vi "GEA2 Script_Parse ERD Read.vi"(0 "Data":string, 11 "Error In":errorcluster) -> (2 "Expected Responses":string[](array[string]), 4 "GEA Inputs":T1 {"Destination" format="%.0x"; "Source" format="%.0x"}, 8 "Read ERD List":T2(array[cluster]) {"ERD Number" format="%.0x"}, 15 "Error Out":errorcluster)   [LabVIEW 2023]
uses:
  LabVIEW GEA2 Toolkit/GEA3/type defs/Source_Destination.ctl
  LabVIEW GEA2 Toolkit/GEA3/type defs/ERD Read Data In.ctl
  <vilib>/regexp/Match Regular Expression.xnode
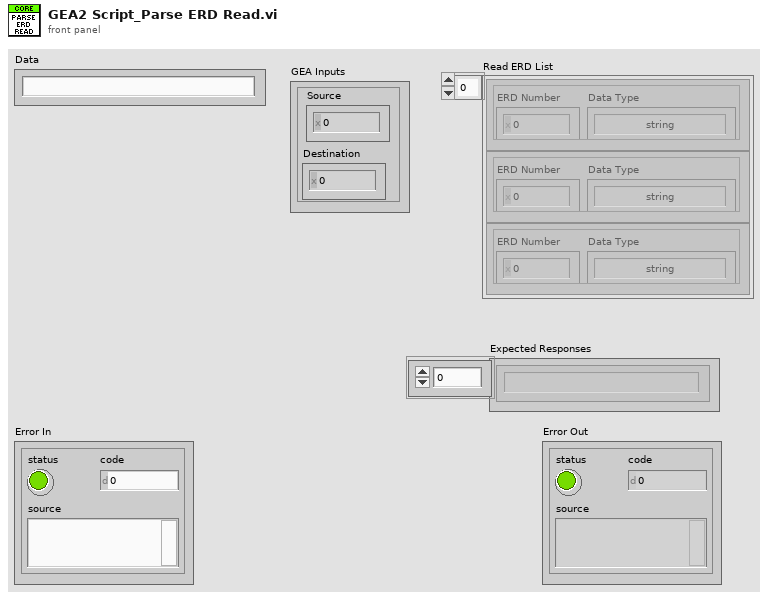
[diagram p1: front panel]
types:
  T1 = typedef "Source_Destination.ctl" = cluster{"Source":u8, "Destination":u8}
  T2 = cluster{"ERD Number":u16, "Data Type":enum16{"string", "boolean", "uint8_t", "uint16_t", "uint32_t", "uint64_t", "int8_t", "int16_t", "int32_t", "int64_t"}}[]
  T3 = typedef "ERD Read Data In.ctl" = cluster{"ERD Number":u16, "Data Type":enum16{"string", "boolean", "uint8_t", "uint16_t", "uint32_t", "uint64_t", "int8_t", "int16_t", "int32_t", "int64_t"}}
  T4 = enum16{"string", "boolean", "uint8_t", "uint16_t", "uint32_t"}
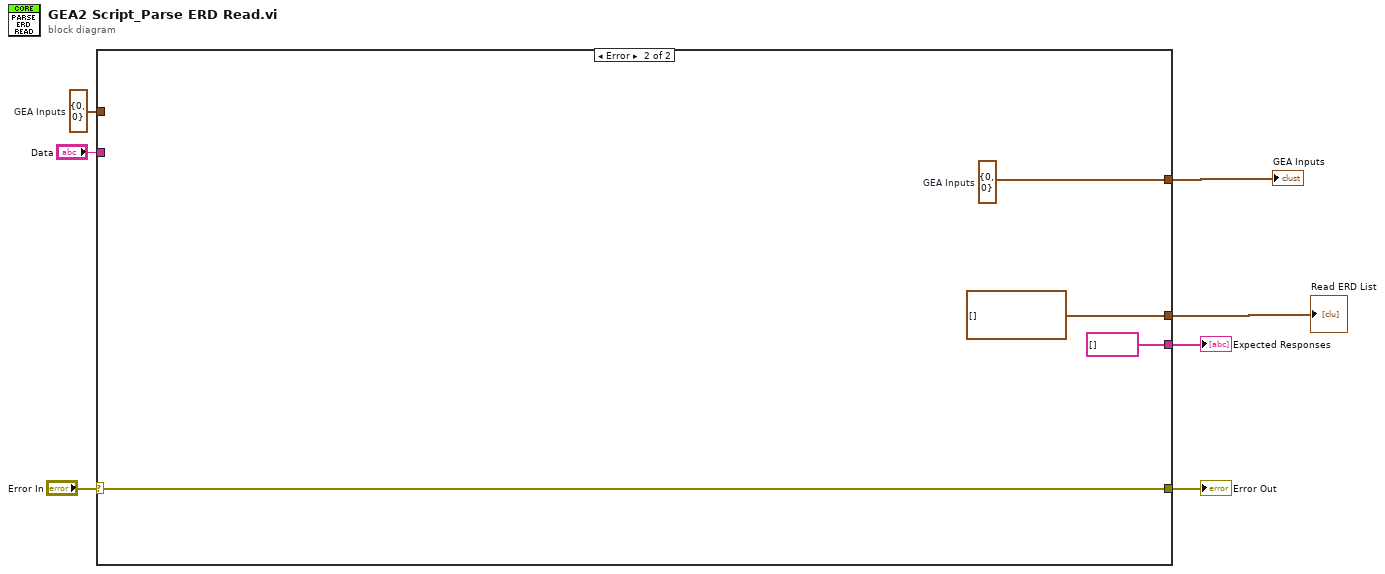
[diagram p0: block diagram]
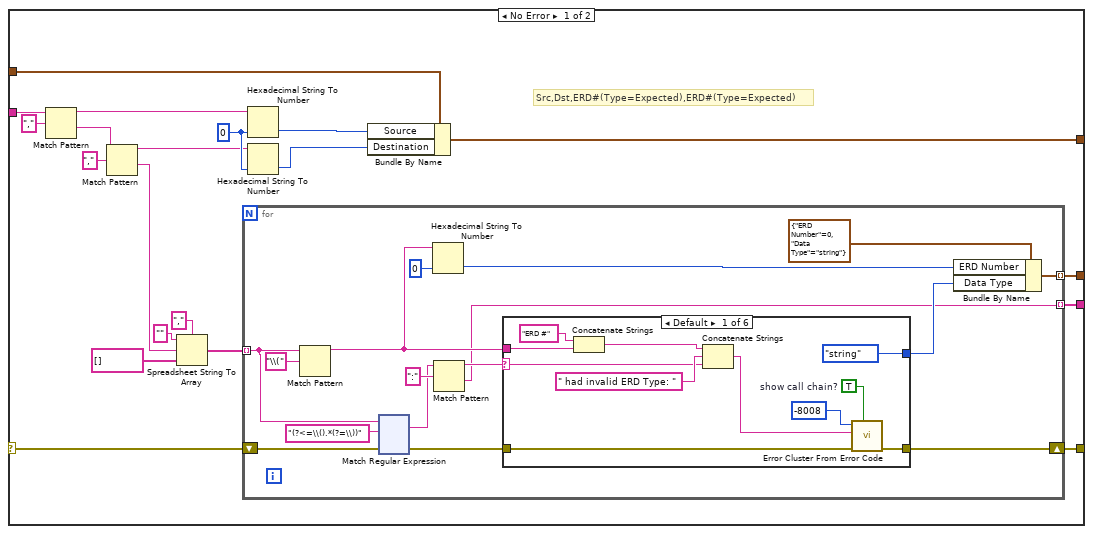
[diagram p2: hidden frame]
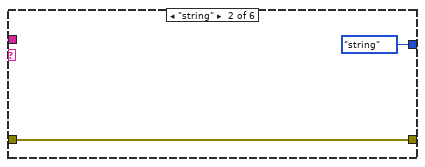
[diagram p3: hidden frame]
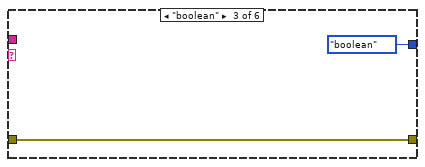
[diagram p4: hidden frame]
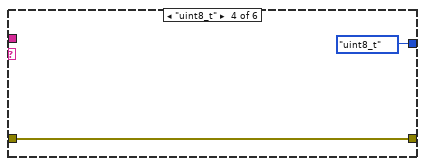
[diagram p5: hidden frame]
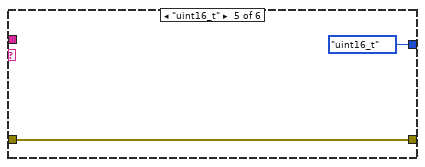
[diagram p6: hidden frame]
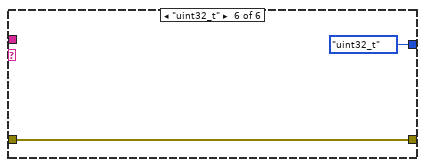
[diagram p7: hidden frame]
diagram:
  w6 = cluster{"Source":u8, "Destination":u8} {"Source"=0, "Destination"=0}  # GEA Inputs
  n1 = case shown="Error" "Error In" {
    selector: "Error In" -> [w16 w185]
    tunnel: "Data" -> [w27 _]
    tunnel: w6 -> [w18 _]
    tunnel: [w17 w182] -> w1
    tunnel: [w15 w185] -> w4
    tunnel: [w9 T2 []] -> w2
    tunnel: [w8 string[] []] -> w3
    frame No Error {
      w21 = u8 0
      # "Src,Dst,ERD#(Type=Expected),ERD#(Type=Expected)"
      n2 = Match Pattern(string=w27, regular expression=",") -> (before substring=w24:string, after substring=w23:string)  [unwired: 1 in, 2 out]
      n3 = Match Pattern(string=w23, regular expression=",") -> (before substring=w20:string, after substring=w13:string)  [unwired: 1 in, 2 out]
      n4 = Spreadsheet String To Array(delimiter (Tab)=",", format string="", spreadsheet string=w13, array type (2D Dbl)=string[] []) -> (array=w11:string[])
      n5 = for {
        tunnel: [w40] -> w9 mode=indexing
        shift-right: [w37] -> w15
        shift-left: w16 -> [w32]
        tunnel: w11 -> [w31] mode=indexing
        tunnel: [w29] -> w8 mode=indexing
        n6 = Match Pattern(string=w31, regular expression="\\(") -> (before substring=w35:string)  [unwired: 1 in, 3 out]
        n7 = xnode "Match Regular Expression"("input string"=w31, "regular expression"="(?<=\\().*(?=\\))", "error in"=w32) -> ("whole match"=w30:string, "error out"=w33:errorcluster)  [unwired: 3 in, 3 out]
        n8 = Hexadecimal String To Number(string=w35, default (0uL)=u16 0 ("ERD Number")) -> (number=w42:u16)  [unwired: 1 in, 1 out]
        n9 = Match Pattern(string=w30, regular expression=":") -> (before substring=w36:string, after substring=w29:string)  [unwired: 1 in, 2 out]
        n10 = case shown="Default" w36 {
          selector: w36 -> [w165 _ _ _ _ _]
          tunnel: [T4."string" ("Data Type") T4."string" ("Data Type") T4."boolean" ("Data Type") T4."uint8_t" ("Data Type") T4."uint16_t" ("Data Type") T4."uint32_t" ("Data Type")] -> w38
          tunnel: w33 -> [w170 w172 w174 w176 w178 w180]
          tunnel: [w169 w172 w174 w176 w178 w180] -> w37
          tunnel: w35 -> [w162 _ _ _ _ _]
          frame Default {
            w167 = TRUE  # show call chain?
            n11 = Concatenate Strings("ERD #", w162) -> (w161:string)
            n12 = Concatenate Strings(w161, " had invalid ERD Type: " ("error message (\"\")"), w165) -> (w164:string)
            n13 = call <vilib>:"Error Cluster From Error Code.vi"("show call chain? (False)"=w167, "error in (no error)"=w170, "error message (\"\")"=w164, "error code (0)"=-8008) -> ("error out"=w169:errorcluster)  [unwired: 5 in]
          }
          frame "string" {
          }
          frame "boolean" {
          }
          frame "uint8_t" {
          }
          frame "uint16_t" {
          }
          frame "uint32_t" {
          }
        }
        n14 = Bundle By Name(cluster=T3 {"ERD Number"=0, "Data Type"=enum."string"} ("ERD Read Data In"), "ERD Number"=w42, "Data Type"=w38) -> (w40:T3)
      }
      n15 = Hexadecimal String To Number(string=w24, default (0uL)=w21) -> (number=w22:u8)  [unwired: 1 in, 1 out]
      n16 = Hexadecimal String To Number(string=w20, default (0uL)=w21) -> (number=w19:u8)  [unwired: 1 in, 1 out]
      n17 = Bundle By Name(cluster=w18, "Source"=w22, "Destination"=w19) -> (w17:cluster{"Source":u8, "Destination":u8})
    }
    frame Error {
      w182 = cluster{"Source":u8, "Destination":u8} {"Source"=0, "Destination"=0}  # GEA Inputs
    }
  }
  "Error Out" <- w4
  "Expected Responses" <- w3
  "Read ERD List" <- w2
  "GEA Inputs" <- w1
